vi "T_step_initial_VTI.vi"(11 "Current Step Setpoint":dbl) -> ()   [LabVIEW 2019]
uses:
  Global/Global Variables/global.vi
  Global/Global Variables/Data_Display_global.vi
  Monitors/Utility/Monitor Communication/sub-vis/VTI_Open_Queue.vi
  Monitors/Utility/Monitor Communication/sub-vis/VTI_Queue_Commands.vi
  Instrument_Setup.vi
  <vilib>/Analysis/NI_AALBase.lvlib
  <vilib>/Analysis/NI_AALPro.lvlib
panel:
  out "Numeric 3":dbl format="%#_13g"
  out "Numeric 2":dbl format="%#_13g"
  out "XY Graph":T1(graph)
  out "Array":dbl[](array[numeric])
  out "Numeric":dbl format="%#_13g"
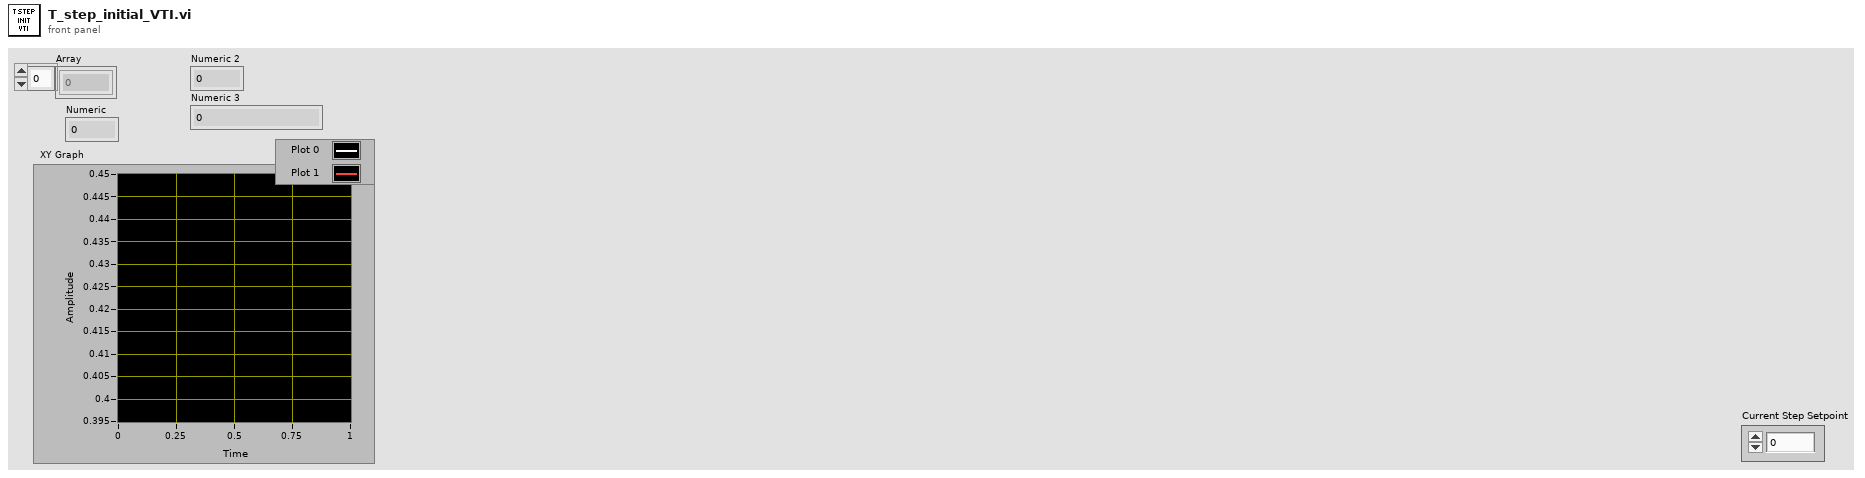
[diagram p1: front panel]
types:
  T1 = cluster{"Plot1":dbl[], "Best Linear Fit":dbl[]}[]
  T2 = typedef "VTI-cluster.ctl" = cluster{"Temperatur (K)":dbl, "Setpoint (K)":dbl, "Rate (K/min)":dbl, "Heater (%)":dbl, "NV (%)":dbl, "Heater Manual":bool, "NV Manual":bool, "Go to Set":bool, "Pressure":dbl, "Heater SP":dbl, "Valid?":bool, "Set Heater SP":bool, "Set NV SP":bool, "Heater (%) Display":dbl, "NV (%) Display":dbl, "NV Setpoint":dbl, "Change Heater Status":bool, "Change NV Status":bool, "Sample 3":dbl, "Sample 2":dbl, "Sweep-State":bool, "Set Auto PID":bool, "Auto PID":bool, "Stopp":bool, "Setpoint-Sweep":dbl}
  T3 = typedef "VTI-control.ctl" = cluster{"Set VTI SP":bool, "Change NV Status":bool, "Set NV Setpoint":bool, "Change Heater Status":bool, "Set Heater Setpoint":bool, "Setpoint (K)":dbl, "Rate (K/min)":dbl, "Setpoint Heater":dbl, "Setpoint NV":dbl, "Change Auto PID":bool, "Stop Sweep":bool}
  T4 = typedef "LS350-cluster.ctl" = cluster{"Setpoint":dbl, "Heater Output":dbl, "Setpoint control":dbl, "Enable Setpoint":bool, "LS350 T1":dbl, "LS350 T2":dbl, "LS350 T3":dbl, "LS350 T4":dbl, "LS350 R1":dbl, "LS350 R2":dbl, "LS350 R3":dbl, "LS350 R4":dbl}
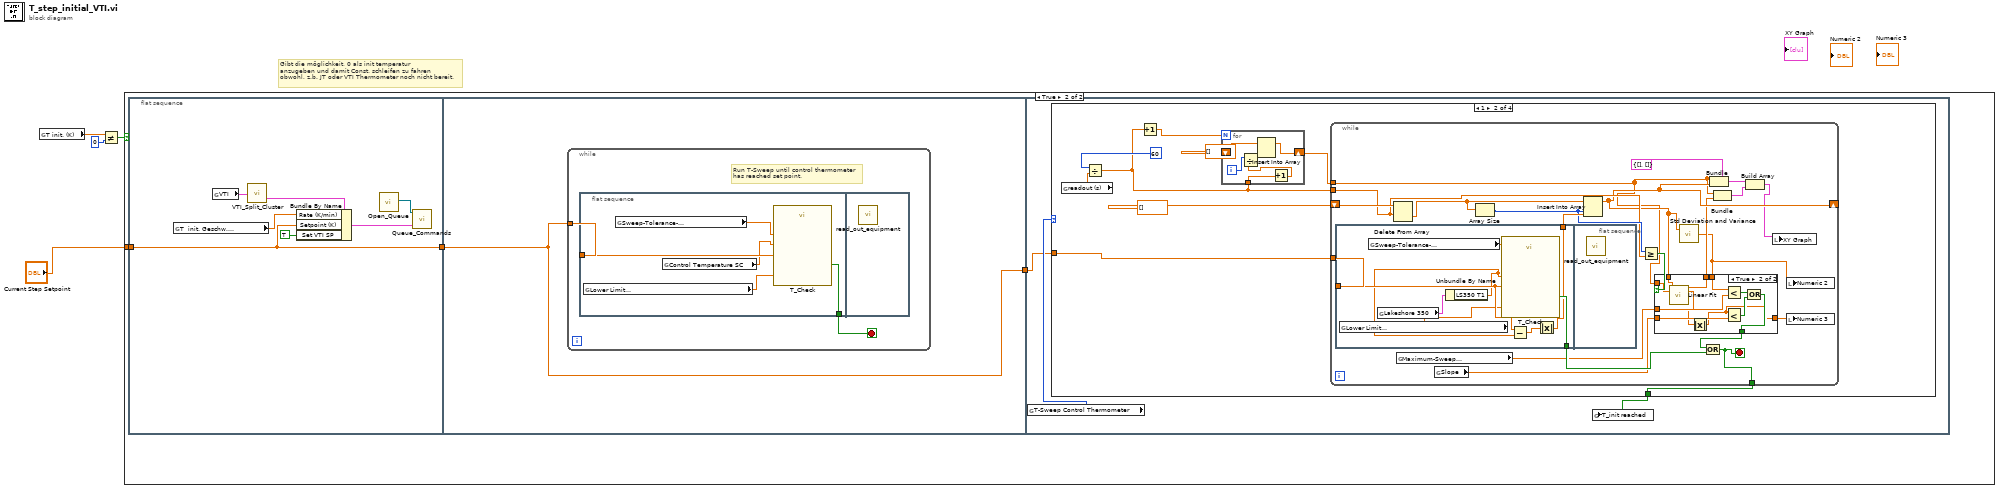
[diagram p0: block diagram]
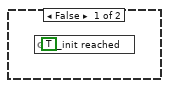
[diagram p2: hidden frame]
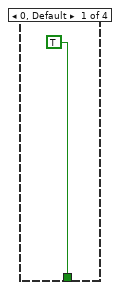
[diagram p3: hidden frame]
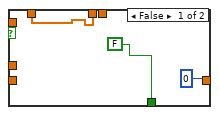
[diagram p4: hidden frame]
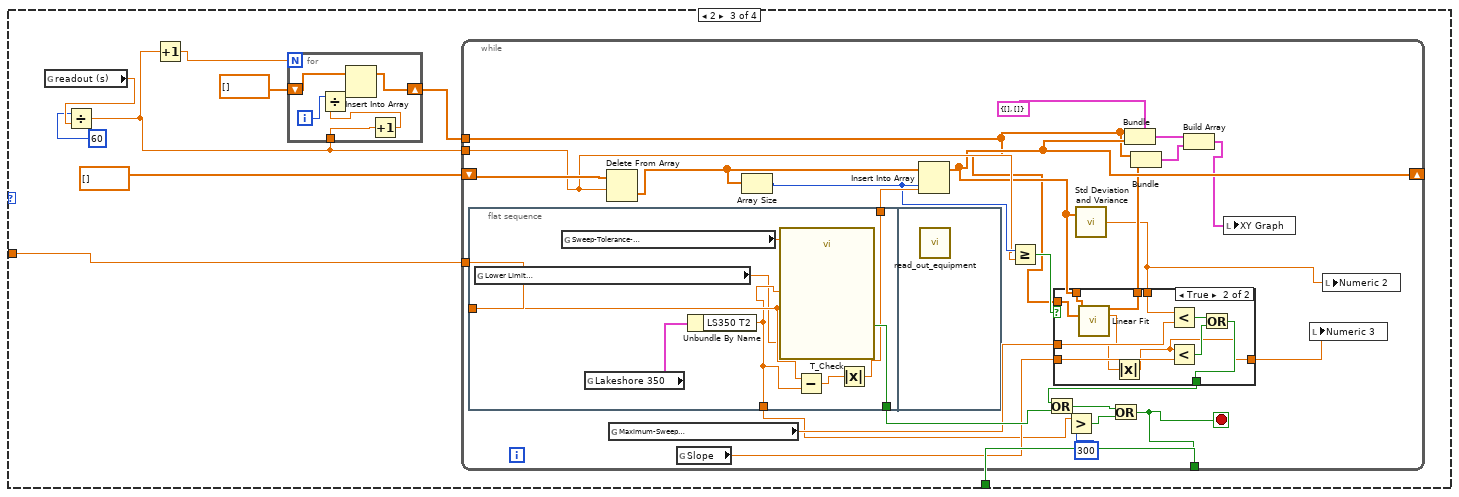
[diagram p5: hidden frame]
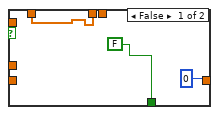
[diagram p6: hidden frame]
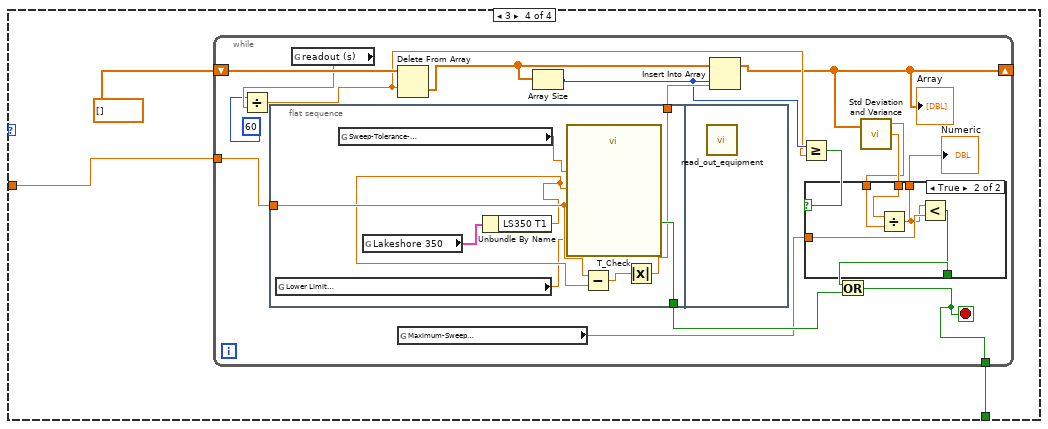
[diagram p7: hidden frame]
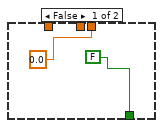
[diagram p8: hidden frame]
diagram:
  # "Gibt die möglichkeit, 0 als init temperatur \nanzugeben und damit Const. schleifen zu fahren\nobwohl, z.b. JT oder VTI Thermometer noch nicht bereit."
  n1 = global read "global.vi" "T init. (K)"() -> (w4:dbl)
  n2 = Not Equal?(x=w4, y=0) -> (x != y?=w2:bool)
  n3 = case shown="True" w2 {
    tunnel: "Current Step Setpoint" -> [_ w6]
    frame False {
      n4 = global write "Data_Display_global.vi" "T_init reached"(TRUE) -> ()
    }
    frame True {
      n5 = flat-sequence {
        tunnel: [w9] -> w8
        tunnel: w6 -> [w9]
        tunnel: w8 -> [w16]
        tunnel: [w16] -> w7
        tunnel: w7 -> [w25]
        frame #0 {
          n6 = global read "global.vi" "T  init. Geschw. \n(K/min)"() -> (w15:dbl)
          n7 = global read "Data_Display_global.vi" "VTI"() -> (w13:T2)
          n8 = call "VTI_Split_Cluster.vi"("VTI"=w13) -> ("VTI Control"=w12:T3)  [unwired: 1 out]
          n9 = Bundle By Name(cluster=w12, "Rate (K/min)"=w15, "Setpoint (K)"=w9, "Set VTI SP"=TRUE) -> (w11:T3)
          n10 = call-poly "Open_Queue.vi"() -> ("queue out"=w14:refnum<queue>)  [unwired: 10 in, 1 out]
          n11 = call-poly "Queue_Commands.vi"("VTI Control"=w11, "20TVTI Queue"=w14) -> ()  [unwired: 1 in, 1 out]
        }
        frame #1 {
          n12 = while {
            tunnel: w16 -> [w18]
            stop <- w17 stop-if-true
            # "Run T-Sweep until control thermometer\nhas reached set point."
            n13 = flat-sequence {
              tunnel: w18 -> [w21]
              tunnel: [w22] -> w17
              frame #0 {
                n14 = global read "Instrument_Setup.vi" "Lower Limit\nSweep-Tolerance-\nTemperature (K)"() -> (w19:dbl)
                n15 = global read "Instrument_Setup.vi" "Sweep-Tolerance-\nTemperature (%)"() -> (w23:dbl)
                n16 = global read "Data_Display_global.vi" "Control Temperature SC"() -> (w20:dbl)
                n17 = call "T_Check.vi"("Lower Limit Sweep\nTolerance (K)"=w19, "T_target (K)"=w21, "Sweep\nTolerance %"=w23, "T_in"=w20) -> ("= T target"=w22:bool)
              }
              frame #1 {
                n18 = call "read_out_equipment.vi"() -> ()  [unwired: 1 in]
              }
            }
          }
        }
        frame #2 {
          n19 = global read "Instrument_Setup.vi" "T-Sweep Control Thermometer"() -> (w26:u16)
          n20 = case shown="1" w26 {
            tunnel: w25 -> [_ w35 w93 w149]
            tunnel: [TRUE w34 w92 w148] -> w24
            frame 0, Default {
            }
            frame 1 {
              n21 = global read "Instrument_Setup.vi" "readout (s)"() -> (w33:dbl)
              n22 = Divide(x=60, y=w33) -> (x/y=w29:dbl)
              n23 = Increment(x=w29) -> (x+1=w28:dbl)
              n24 = for {
                N: w28 -> [_]
                shift-right: [w39] -> w30
                shift-left: dbl[] [] -> [w42]
                tunnel: w29 -> [w38]
                i -> [w41]
                n25 = Increment(x=w38) -> (x+1=w37:dbl)
                n26 = Divide(x=w41, y=w37) -> (x/y=w40:dbl)
                n27 = Insert Into Array(array=w42, new element=w40) -> (w39:dbl[])  [unwired: 1 in]
              }
              n28 = while {
                tunnel: w35 -> [w63]
                shift-right: [w50] -> _
                shift-left: dbl[] [] -> [w62]
                tunnel: [w55] -> w34
                tunnel: w29 -> [w51]
                tunnel: w30 -> [w49]
                stop <- w55 stop-if-true
                n29 = flat-sequence {
                  tunnel: w63 -> [w84]
                  tunnel: [w81] -> w61
                  tunnel: [w85] -> w60
                  frame #0 {
                    n30 = global read "Instrument_Setup.vi" "Lower Limit\nSweep-Tolerance-\nTemperature (K)"() -> (w78:dbl)
                    n31 = global read "Instrument_Setup.vi" "Sweep-Tolerance-\nTemperature (%)"() -> (w79:dbl)
                    n32 = global read "Data_Display_global.vi" "Lakeshore 350"() -> (w80:T4)
                    n33 = Unbundle By Name(w80) -> ("LS350 T1"=w83:dbl)
                    n34 = call "T_Check.vi"("Lower Limit Sweep\nTolerance (K)"=w78, "T_target (K)"=w84, "Sweep\nTolerance %"=w79, "T_in"=w83) -> ("= T target"=w85:bool)
                    n35 = Subtract(x=w84, y=w83) -> (x-y=w82:dbl)
                    n36 = Absolute Value(x=w82) -> (abs(x)=w81:dbl)
                  }
                  frame #1 {
                    n37 = call "read_out_equipment.vi"() -> ()  [unwired: 1 in]
                  }
                }
                n38 = Delete From Array(array=w62, length=w51) -> (deleted portion=w58:dbl[])  [unwired: 1 in, 1 out]
                n39 = global read "Instrument_Setup.vi" "Maximum-Sweep\nSettle %/min"() -> (w56:dbl)
                n40 = global read "Instrument_Setup.vi" "Slope"() -> (w53:dbl)
                n41 = Array Size(array=w58) -> (size(s)=w52:i32)
                n42 = Insert Into Array(array=w58, index=w52, new element=w61) -> (w50:dbl[])
                n43 = Greater Or Equal?(x=w52, y=w51) -> (x >= y?=w57:bool)
                n44 = call <vilib>:"Std Deviation and Variance.vi"("X"=w50) -> ("standard deviation"=w44:dbl)  [unwired: 1 in, 2 out]
                n45 = case shown="True" w57 {
                  tunnel: w44 -> [_ w76]
                  tunnel: [FALSE w69] -> w59
                  tunnel: w56 -> [_ w77]
                  tunnel: w49 -> [_ w74]
                  tunnel: w50 -> [w65 w73]
                  tunnel: [w65 w72] -> w48
                  tunnel: w53 -> [_ w71]
                  tunnel: [0 w67] -> w45
                  frame False {
                  }
                  frame True {
                    n46 = call <vilib>:"Linear Fit.vi"("Y"=w73, "X"=w74) -> ("Best Linear Fit"=w72:dbl[], "slope"=w68:dbl)  [unwired: 9 in, 3 out]
                    n47 = Absolute Value(x=w68) -> (abs(x)=w67:dbl)
                    n48 = Less?(x=w76, y=w77) -> (x < y?=w75:bool)
                    n49 = Less?(x=w67, y=w71) -> (x < y?=w70:bool)
                    n50 = Or(x=w75, y=w70) -> (x .or. y?=w69:bool)
                  }
                }
                n51 = Or(x=w59, y=w60) -> (x .or. y?=w55:bool)
                n52 = Bundle(cluster=cluster{"Plot1":dbl[], "Plot 2":dbl[]} {"Plot1"=[], "Plot 2"=[]}, "Plot1"=w49, "Plot 2"=w50) -> (w47:cluster{"Plot1":dbl[], "Plot 2":dbl[]})
                n53 = Bundle(w49, "Best Linear Fit"=w48) -> (w46:cluster{dbl[], "Best Linear Fit":dbl[]})  [unwired: 1 in]
                n54 = Build Array(w47, w46) -> (w43:T1)
                n55 = local write "XY Graph"(w43) -> ()
                n56 = local write "Numeric 2"(w44) -> ()
                n57 = local write "Numeric 3"(w45) -> ()
              }
            }
            frame 2 {
              n58 = global read "Instrument_Setup.vi" "readout (s)"() -> (w91:dbl)
              n59 = Divide(x=60, y=w91) -> (x/y=w87:dbl)
              n60 = Increment(x=w87) -> (x+1=w86:dbl)
              n61 = for {
                N: w86 -> [_]
                shift-right: [w97] -> w88
                shift-left: dbl[] [] -> [w100]
                tunnel: w87 -> [w96]
                i -> [w99]
                n62 = Increment(x=w96) -> (x+1=w95:dbl)
                n63 = Divide(x=w99, y=w95) -> (x/y=w98:dbl)
                n64 = Insert Into Array(array=w100, new element=w98) -> (w97:dbl[])  [unwired: 1 in]
              }
              n65 = while {
                tunnel: w93 -> [w125]
                shift-right: [w113] -> _
                shift-left: dbl[] [] -> [w124]
                tunnel: [w101] -> w92
                tunnel: w87 -> [w114]
                tunnel: w88 -> [w112]
                stop <- w101 stop-if-true
                n66 = flat-sequence {
                  tunnel: w125 -> [w146]
                  tunnel: [w144] -> w123
                  tunnel: [w147] -> w122
                  tunnel: [w142] -> w105
                  frame #0 {
                    n67 = global read "Instrument_Setup.vi" "Lower Limit\nSweep-Tolerance-\nTemperature (K)"() -> (w140:dbl)
                    n68 = global read "Instrument_Setup.vi" "Sweep-Tolerance-\nTemperature (%)"() -> (w141:dbl)
                    n69 = global read "Data_Display_global.vi" "Lakeshore 350"() -> (w143:T4)
                    n70 = Unbundle By Name(w143) -> ("LS350 T2"=w142:dbl)
                    n71 = call "T_Check.vi"("Lower Limit Sweep\nTolerance (K)"=w140, "T_target (K)"=w146, "Sweep\nTolerance %"=w141, "T_in"=w142) -> ("= T target"=w147:bool)
                    n72 = Subtract(x=w146, y=w142) -> (x-y=w145:dbl)
                    n73 = Absolute Value(x=w145) -> (abs(x)=w144:dbl)
                  }
                  frame #1 {
                    n74 = call "read_out_equipment.vi"() -> ()  [unwired: 1 in]
                  }
                }
                n75 = Delete From Array(array=w124, length=w114) -> (deleted portion=w120:dbl[])  [unwired: 1 in, 1 out]
                n76 = global read "Instrument_Setup.vi" "Maximum-Sweep\nSettle %/min"() -> (w118:dbl)
                n77 = global read "Instrument_Setup.vi" "Slope"() -> (w116:dbl)
                n78 = Array Size(array=w120) -> (size(s)=w115:i32)
                n79 = Insert Into Array(array=w120, index=w115, new element=w123) -> (w113:dbl[])
                n80 = Greater Or Equal?(x=w115, y=w114) -> (x >= y?=w119:bool)
                n81 = Greater?(x=w105, y=300) -> (0:w103:bool)
                n82 = call <vilib>:"Std Deviation and Variance.vi"("X"=w113) -> ("standard deviation"=w107:dbl)  [unwired: 1 in, 2 out]
                n83 = case shown="True" w119 {
                  tunnel: w107 -> [_ w138]
                  tunnel: [FALSE w131] -> w121
                  tunnel: w118 -> [_ w139]
                  tunnel: w112 -> [_ w136]
                  tunnel: w113 -> [w127 w135]
                  tunnel: [w127 w134] -> w111
                  tunnel: w116 -> [_ w133]
                  tunnel: [0 w129] -> w106
                  frame False {
                  }
                  frame True {
                    n84 = call <vilib>:"Linear Fit.vi"("Y"=w135, "X"=w136) -> ("Best Linear Fit"=w134:dbl[], "slope"=w130:dbl)  [unwired: 9 in, 3 out]
                    n85 = Absolute Value(x=w130) -> (abs(x)=w129:dbl)
                    n86 = Less?(x=w138, y=w139) -> (x < y?=w137:bool)
                    n87 = Less?(x=w129, y=w133) -> (x < y?=w132:bool)
                    n88 = Or(x=w137, y=w132) -> (x .or. y?=w131:bool)
                  }
                }
                n89 = Or(x=w121, y=w122) -> (x .or. y?=w102:bool)
                n90 = Or(x=w102, y=w103) -> (x .or. y?=w101:bool)
                n91 = Bundle(cluster=cluster{"Plot1":dbl[], "Plot 2":dbl[]} {"Plot1"=[], "Plot 2"=[]}, "Plot1"=w112, "Plot 2"=w113) -> (w110:cluster{"Plot1":dbl[], "Plot 2":dbl[]})
                n92 = Bundle(w112, "Best Linear Fit"=w111) -> (w109:cluster{dbl[], "Best Linear Fit":dbl[]})  [unwired: 1 in]
                n93 = Build Array(w110, w109) -> (w108:T1)
                n94 = local write "XY Graph"(w108) -> ()
                n95 = local write "Numeric 3"(w106) -> ()
                n96 = local write "Numeric 2"(w107) -> ()
              }
            }
            frame 3 {
              n97 = while {
                tunnel: w149 -> [w167]
                shift-right: [w153] -> _
                shift-left: dbl[] [] -> [w166]
                tunnel: [w151] -> w148
                stop <- w151 stop-if-true
                n98 = flat-sequence {
                  tunnel: w167 -> [w181]
                  tunnel: [w178] -> w165
                  tunnel: [w182] -> w163
                  frame #0 {
                    n99 = global read "Instrument_Setup.vi" "Lower Limit\nSweep-Tolerance-\nTemperature (K)"() -> (w175:dbl)
                    n100 = global read "Instrument_Setup.vi" "Sweep-Tolerance-\nTemperature (%)"() -> (w176:dbl)
                    n101 = global read "Data_Display_global.vi" "Lakeshore 350"() -> (w177:T4)
                    n102 = Unbundle By Name(w177) -> ("LS350 T1"=w180:dbl)
                    n103 = call "T_Check.vi"("Lower Limit Sweep\nTolerance (K)"=w175, "T_target (K)"=w181, "Sweep\nTolerance %"=w176, "T_in"=w180) -> ("= T target"=w182:bool)
                    n104 = Subtract(x=w181, y=w180) -> (x-y=w179:dbl)
                    n105 = Absolute Value(x=w179) -> (abs(x)=w178:dbl)
                  }
                  frame #1 {
                    n106 = call "read_out_equipment.vi"() -> ()  [unwired: 1 in]
                  }
                }
                n107 = global read "Instrument_Setup.vi" "readout (s)"() -> (w157:dbl)
                n108 = Divide(x=60, y=w157) -> (x/y=w155:dbl)
                n109 = Delete From Array(array=w166, length=w155) -> (deleted portion=w161:dbl[])  [unwired: 1 in, 1 out]
                n110 = global read "Instrument_Setup.vi" "Maximum-Sweep\nSettle %/min"() -> (w154:dbl)
                n111 = Array Size(array=w161) -> (size(s)=w160:i32)
                n112 = Insert Into Array(array=w161, index=w160, new element=w165) -> (w153:dbl[])
                "Array" <- w153
                n113 = Greater Or Equal?(x=w160, y=w155) -> (x >= y?=w159:bool)
                n114 = call <vilib>:"Std Deviation and Variance.vi"("X"=w153) -> ("mean"=w158:dbl, "standard deviation"=w164:dbl)  [unwired: 1 in, 1 out]
                n115 = case shown="True" w159 {
                  tunnel: w164 -> [_ w174]
                  tunnel: [FALSE w172] -> w162
                  tunnel: w158 -> [_ w173]
                  tunnel: w154 -> [_ w171]
                  tunnel: [0.0 w170] -> w152
                  frame False {
                  }
                  frame True {
                    n116 = Divide(x=w174, y=w173) -> (x/y=w170:dbl)
                    n117 = Less?(x=w170, y=w171) -> (x < y?=w172:bool)
                  }
                }
                "Numeric" <- w152
                n118 = Or(x=w162, y=w163) -> (x .or. y?=w151:bool)
              }
            }
          }
          n119 = global write "Data_Display_global.vi" "T_init reached"(w24) -> ()
        }
      }
    }
  }
